vi "TouchPanel.Main.vi"(11 "VI ref":refnum<vi>) -> (1 "Canceled":bool, 2 "Label.Text":string, 3 "control used?":bool)   [LabVIEW 2016]
panel:
  out "Canceled 2":bool
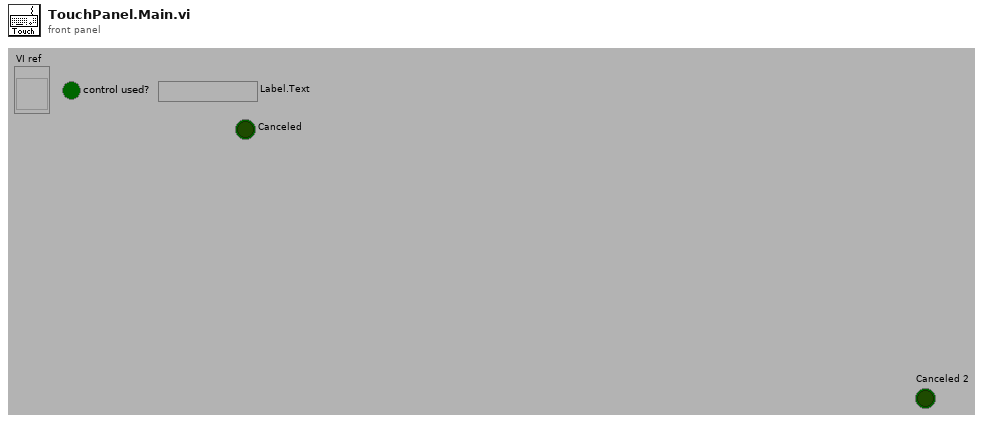
[diagram p1: front panel]
types:
  T1 = typedef "LVNumericRepresentation.ctl" = enum32{"Extended Precision", "Double Precision", "Single Precision", "Long", "Word", "Byte", "Unsigned Long", "Unsigned Word", "Unsigned Byte", "Complex Extended", "Complex Double", "Complex Single", "Quad", "Unsigned Quad", "Fixed-Point"}
  T2 = typedef "LVRowAndColumnTypeDef.ctl" = cluster{"Row":i32, "Column":i32}
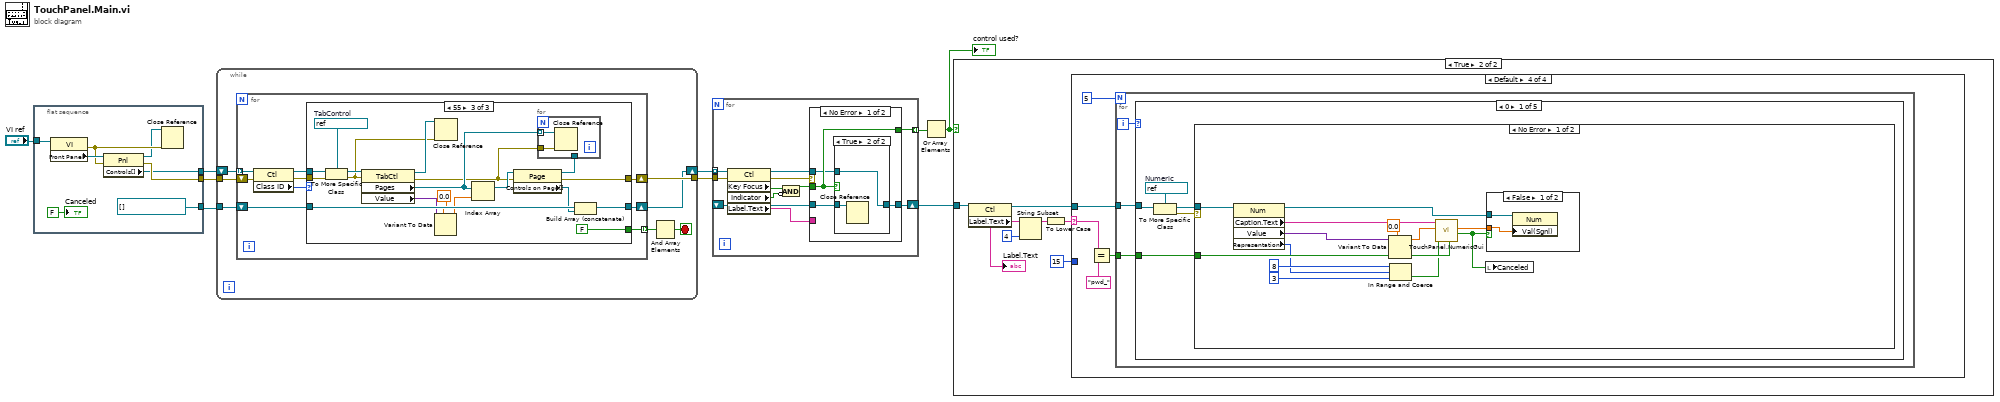
[diagram p0: block diagram]
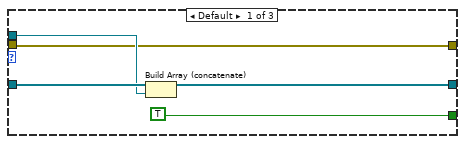
[diagram p2: hidden frame]
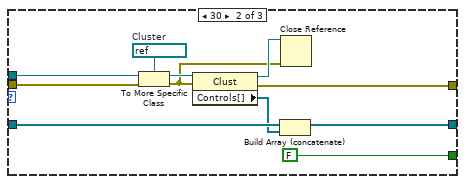
[diagram p3: hidden frame]
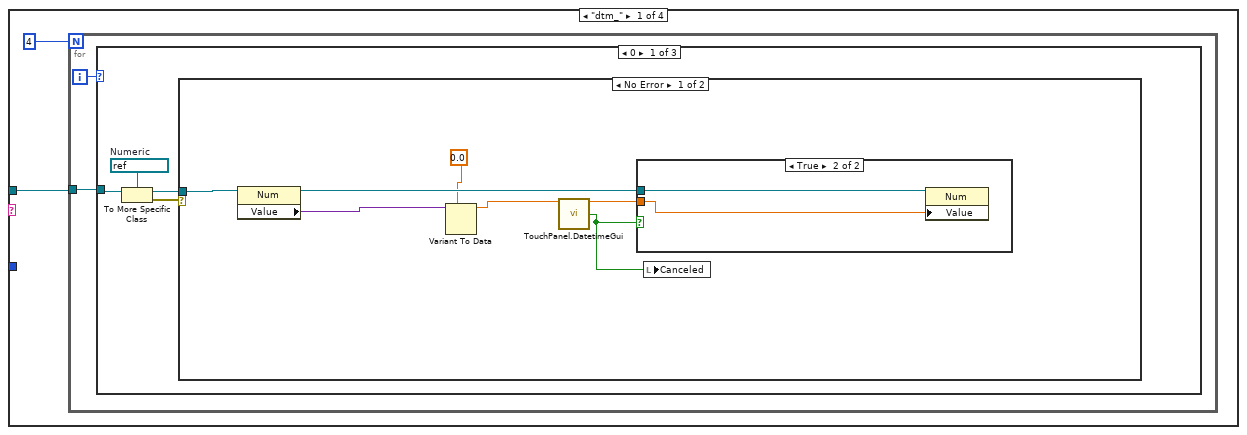
[diagram p5: hidden frame]
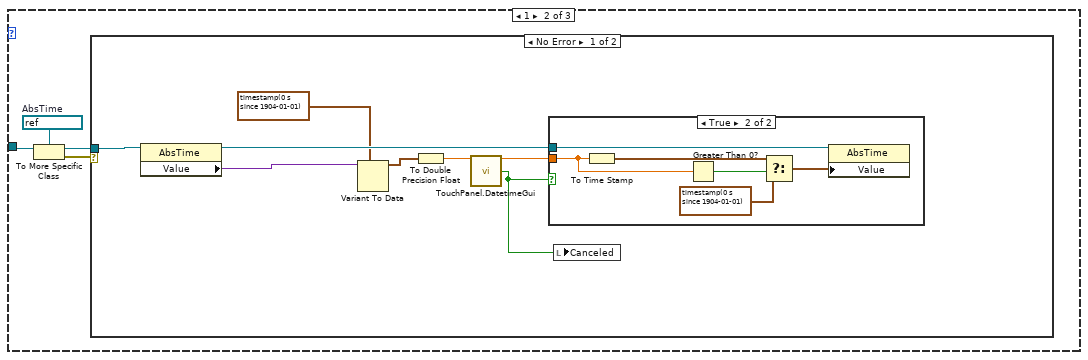
[diagram p8: hidden frame]
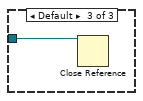
[diagram p11: hidden frame]
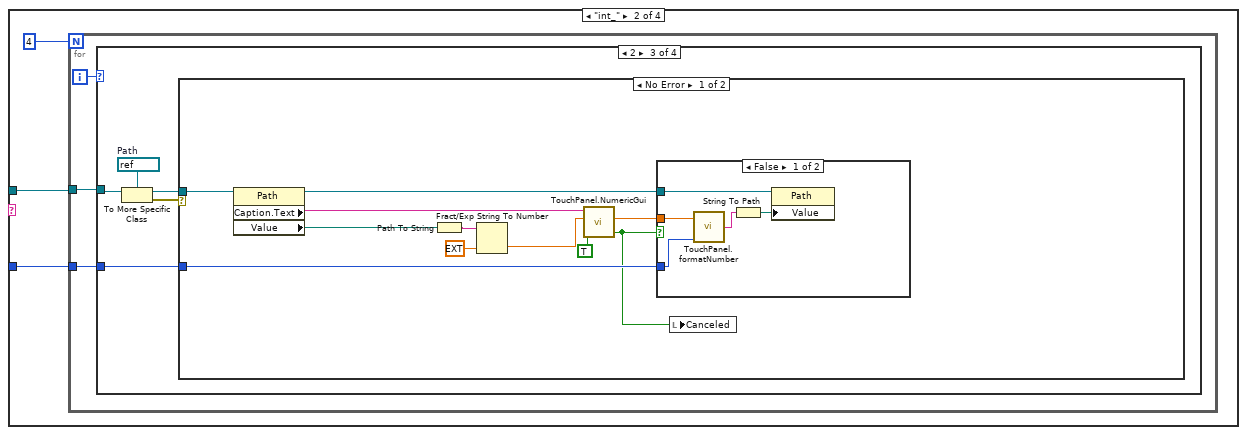
[diagram p12: hidden frame]
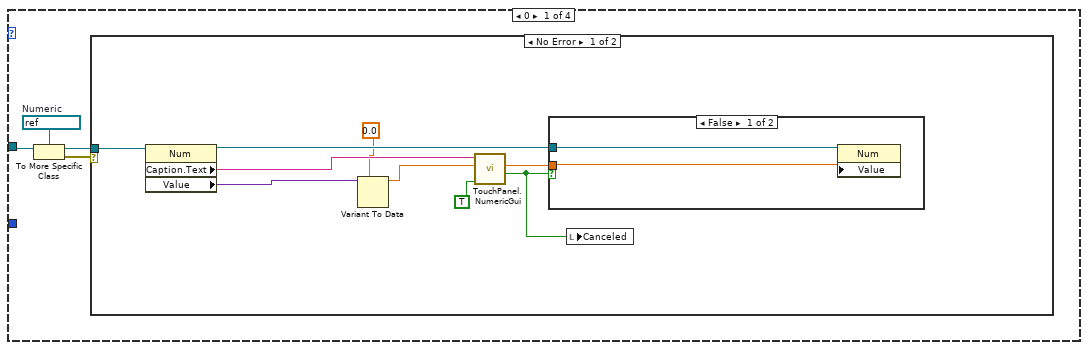
[diagram p13: hidden frame]
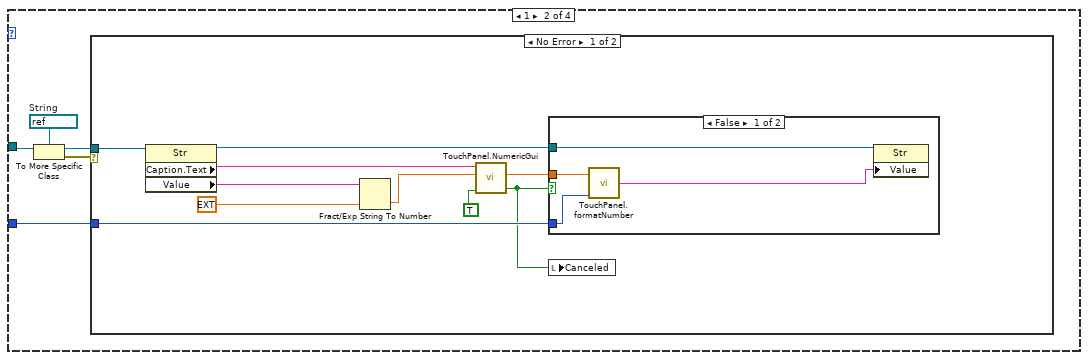
[diagram p16: hidden frame]
diagram:
  n1 = flat-sequence {
    tunnel: [w14] -> w7
    tunnel: [refnum<vi>[] []] -> w5
    tunnel: [w12] -> w4
    tunnel: "VI ref" -> [w11]
    frame #0 {
      n2 = property class="VI"(reference=w11) -> (error out=w16:errorcluster, "Front Panel"=w17:refnum<vi>)  [unwired: 1 in, 1 out]
      n3 = property class="Pnl"(reference=w17, error in=w16) -> (reference out=w15:refnum<vi>, error out=w14:errorcluster, "Controls[]"=w12:refnum<vi>[])
      n4 = Close Reference(reference=w15, error in (no error)=w16) -> ()  [unwired: 1 out]
      "Canceled" <- FALSE ("Canceled")
    }
  }
  n5 = while {
    tunnel: w7 -> [w24]
    tunnel: [w23] -> w6
    tunnel: w5 -> [w22]
    shift-right: [w20] -> w3
    shift-left: w4 -> [w21]
    stop <- w18 stop-if-true
    n6 = for {
      tunnel: w21 -> [w33] mode=indexing
      shift-right: [w27] -> w23
      shift-left: w24 -> [w32]
      shift-right: [w28] -> w20
      shift-left: w22 -> [w29]
      tunnel: [w25] -> w19 mode=indexing
      n7 = property class="Ctl"(reference=w33, error in=w32) -> (reference out=w31:refnum<vi>, error out=w30:errorcluster, "Class ID"=w26:u32)
      n8 = case shown="55" w26 {
        tunnel: w31 -> [w37 w47 w66]
        tunnel: w30 -> [w35 w46 w65]
        tunnel: w29 -> [w38 w43 w61]
        tunnel: [w36 w41 w60] -> w28
        tunnel: [w35 w40 w59] -> w27
        tunnel: [TRUE FALSE FALSE] -> w25
        frame Default {
          n9 = Build Array (concatenate)(w38, w37) -> (w36:refnum<vi>[])
        }
        frame 30 {
          w48 = refnum<vi> refnum  # Cluster
          n10 = To More Specific Class(target class=w48, reference=w47, error in=w46) -> (specific class reference=w49:refnum<vi>, error out=w44:errorcluster)
          n11 = property class="Clust"(reference=w49, error in=w44) -> (reference out=w45:refnum<vi>, error out=w40:errorcluster, "Controls[]"=w42:refnum<vi>[])
          n12 = Build Array (concatenate)(w43, w42) -> (w41:refnum<vi>[])
          n13 = Close Reference(reference=w45, error in (no error)=w44) -> ()  [unwired: 1 out]
        }
        frame 55 {
          w62 = refnum<vi> refnum  # TabControl
          n14 = To More Specific Class(target class=w62, reference=w66, error in=w65) -> (specific class reference=w67:refnum<vi>, error out=w63:errorcluster)
          n15 = property class="TabCtl"(reference=w67, error in=w63) -> (reference out=w64:refnum<vi>, error out=w51:errorcluster, "Pages"=w52:refnum<vi>[], "Value"=w57:variant)
          n16 = Variant To Data(type=0.0 ("value"), Variant=w57) -> (data=w55:dbl)  [unwired: 1 in, 1 out]
          n17 = Close Reference(reference=w64, error in (no error)=w63) -> ()  [unwired: 1 out]
          n18 = Index Array(array=w52, index=w55) -> (element=w54:refnum<vi>)
          n19 = property class="Page"(reference=w54, error in=w51) -> (reference out=w50:refnum<vi>, error out=w59:errorcluster, "Controls on Page[]"=w53:refnum<vi>[])
          n20 = for {
            tunnel: w52 -> [w69] mode=indexing
            tunnel: w51 -> [w68]
            tunnel: w50 -> [_]
            n21 = Close Reference(reference=w69, error in (no error)=w68) -> ()  [unwired: 1 out]
          }
          n22 = Build Array (concatenate)(w61, w53) -> (w60:refnum<vi>[])
        }
      }
    }
    n23 = And Array Elements(Boolean array=w19) -> (logical AND=w18:bool)
  }
  n24 = for {
    tunnel: w3 -> [w80] mode=indexing
    shift-right: [w75] -> w8
    shift-left: _ -> [w77]
    tunnel: w6 -> [w79]
    tunnel: [w74] -> w9 mode=indexing
    n25 = property class="Ctl"(reference=w80, error in=w79) -> (reference out=w78:refnum<vi>, error out=w76:errorcluster, "Key Focus"=w72:bool, "Indicator"=w71:bool, "Label.Text"=w70:string)
    n26 = Compound Arithmetic op=AND(w72, invert w71) -> (w73:bool)
    n27 = case shown="No Error" w76 {
      tunnel: w78 -> [w83 _]
      tunnel: w77 -> [w82 w90]
      tunnel: w73 -> [w84 _]
      tunnel: [w81 w90] -> w75
      tunnel: [w84 FALSE ("Key Focus")] -> w74
      tunnel: w70 -> [_ _]
      frame No Error {
        n28 = case shown="True" w84 {
          tunnel: w83 -> [w86 w87]
          tunnel: w82 -> [w85 w88]
          tunnel: [w85 w87] -> w81
          frame False {
            n29 = Close Reference(reference=w86) -> ()  [unwired: 1 in, 1 out]
          }
          frame True {
            n30 = Close Reference(reference=w88) -> ()  [unwired: 1 in, 1 out]
          }
        }
      }
      frame Error {
      }
    }
  }
  n31 = Or Array Elements(Boolean array=w9) -> (logical OR=w2:bool)
  "control used?" <- w2
  n32 = case shown="True" w2 {
    tunnel: w8 -> [_ w97]
    frame False {
    }
    frame True {
      n33 = property class="Ctl"(reference=w97) -> (reference out=w96:refnum<vi>, "Label.Text"=w91:string)  [unwired: 1 in, 1 out]
      "Label.Text" <- w91
      n34 = String Subset(string=w91, length (rest)=4 ("length (rest)")) -> (substring=w95:string)  [unwired: 1 out]
      n35 = To Lower Case(string=w95) -> (all lower case string=w93:string)
      n36 = case shown="Default" w93 {
        selector: w93 -> [_ _ _ w260]
        tunnel: w96 -> [w98 w135 w197 w262]
        tunnel: i16 15 ("significant digits (6)") -> [_ w134 w196 _]
        frame "dtm_" {
          n37 = for {
            N: 4 -> [_]
            tunnel: w98 -> [w101]
            i -> [w100]
            n38 = case shown="0" w100 {
              tunnel: w101 -> [w102 w115 w133]
              frame 0 {
                w105 = refnum<vi> refnum  # Numeric
                n39 = To More Specific Class(target class=w105, reference=w102) -> (specific class reference=w103:refnum<vi>, error out=w104:errorcluster)  [unwired: 1 in]
                n40 = case shown="No Error" w104 {
                  tunnel: w103 -> [w112 _]
                  frame No Error {
                    n41 = property class="Num"(reference=w112) -> (reference out=w111:refnum<vi>, "Value"=w110:variant)  [unwired: 1 in, 1 out]
                    n42 = Variant To Data(type=0.0 ("value"), Variant=w110) -> (data=w108:dbl)  [unwired: 1 in, 1 out]
                    n43 = call "TouchPanel.DatetimeGui.vi"("num date/time in (now)"=w108) -> ("num date/time out"=w107:dbl, "ok"=w106:bool)  [unwired: 1 in, 12 out]
                    n44 = case shown="True" w106 {
                      tunnel: w111 -> [_ w114]
                      tunnel: w107 -> [_ w113]
                      frame False {
                      }
                      frame True {
                        n45 = property class="Num"(reference=w114, "Value"=w113) -> ()  [unwired: 1 in, 2 out]
                      }
                    }
                    n46 = local write "Canceled"(w106) -> ()
                  }
                  frame Error {
                  }
                }
              }
              frame 1 {
                w118 = refnum<vi> refnum  # AbsTime
                n47 = To More Specific Class(target class=w118, reference=w115) -> (specific class reference=w116:refnum<vi>, error out=w117:errorcluster)  [unwired: 1 in]
                n48 = case shown="No Error" w117 {
                  tunnel: w116 -> [w126 _]
                  frame No Error {
                    n49 = property class="AbsTime"(reference=w126) -> (reference out=w125:refnum<vi>, "Value"=w124:variant)  [unwired: 1 in, 1 out]
                    n50 = Variant To Data(type=timestamp(0 s since 1904-01-01), Variant=w124) -> (data=w123:timestamp)  [unwired: 1 in, 1 out]
                    n51 = To Double Precision Float(number=w123) -> (double precision float=w120:dbl)
                    n52 = call "TouchPanel.DatetimeGui.vi"("num date/time in (now)"=w120) -> ("num date/time out"=w122:dbl, "ok"=w119:bool)  [unwired: 1 in, 12 out]
                    n53 = case shown="True" w119 {
                      tunnel: w125 -> [_ w132]
                      tunnel: w122 -> [_ w128]
                      frame False {
                      }
                      frame True {
                        n54 = To Time Stamp(1:w128) -> (0:w130:timestamp)
                        n55 = Greater Than 0?(x=w128) -> (x > 0?=w131:bool)
                        n56 = Select(t=w130, s=w131, f=timestamp(0 s since 1904-01-01) ("time stamp")) -> (s? t:f=w129:timestamp)
                        n57 = property class="AbsTime"(reference=w132, "Value"=w129) -> ()  [unwired: 1 in, 2 out]
                      }
                    }
                    n58 = local write "Canceled"(w119) -> ()
                  }
                  frame Error {
                  }
                }
              }
              frame Default {
                n59 = Close Reference(reference=w133) -> ()  [unwired: 1 in, 1 out]
              }
            }
          }
        }
        frame "int_" {
          n60 = for {
            N: 4 -> [_]
            tunnel: w135 -> [w139]
            tunnel: w134 -> [w137]
            i -> [w138]
            n61 = case shown="2" w138 {
              tunnel: w139 -> [w140 w157 w176 w195]
              tunnel: w137 -> [_ w155 w174 _]
              frame 0 {
                w143 = refnum<vi> refnum  # Numeric
                n62 = To More Specific Class(target class=w143, reference=w140) -> (specific class reference=w141:refnum<vi>, error out=w142:errorcluster)  [unwired: 1 in]
                n63 = case shown="No Error" w142 {
                  tunnel: w141 -> [w152 _]
                  frame No Error {
                    n64 = property class="Num"(reference=w152) -> (reference out=w151:refnum<vi>, "Caption.Text"=w149:string, "Value"=w150:variant)  [unwired: 1 in, 1 out]
                    n65 = Variant To Data(type=0.0 ("value"), Variant=w150) -> (data=w147:dbl)  [unwired: 1 in, 1 out]
                    n66 = call "TouchPanel.NumericGui.vi"("Integer (F)"=TRUE, "Numeric In"=w147, "Message In"=w149) -> ("Canceled"=w144:bool, "Numeric Out"=w146:ext)  [unwired: 3 in, 4 out]
                    n67 = case shown="False" w144 {
                      tunnel: w151 -> [w154 _]
                      tunnel: w146 -> [w153 _]
                      frame False {
                        n68 = property class="Num"(reference=w154, "Value"=w153) -> ()  [unwired: 1 in, 2 out]
                      }
                      frame True {
                      }
                    }
                    n69 = local write "Canceled"(w144) -> ()
                  }
                  frame Error {
                  }
                }
              }
              frame 1 {
                w156 = refnum<vi> refnum  # String
                n70 = To More Specific Class(target class=w156, reference=w157) -> (specific class reference=w158:refnum<vi>, error out=w159:errorcluster)  [unwired: 1 in]
                n71 = case shown="No Error" w159 {
                  tunnel: w158 -> [w169 _]
                  tunnel: w155 -> [w161 _]
                  frame No Error {
                    n72 = property class="Str"(reference=w169) -> (reference out=w168:refnum<vi>, "Caption.Text"=w165:string, "Value"=w167:string)  [unwired: 1 in, 1 out]
                    n73 = Fract/Exp String To Number(string=w167, default (0 dbl)=ext 0.0 ("default (0 DBL)")) -> (number=w164:ext)  [unwired: 1 in, 2 out]
                    n74 = call "TouchPanel.NumericGui.vi"("Integer (F)"=TRUE, "Numeric In"=w164, "Message In"=w165) -> ("Canceled"=w160:bool, "Numeric Out"=w163:ext)  [unwired: 3 in, 4 out]
                    n75 = case shown="False" w160 {
                      tunnel: w168 -> [w173 _]
                      tunnel: w163 -> [w172 _]
                      tunnel: w161 -> [w170 _]
                      frame False {
                        n76 = call "TouchPanel.formatNumber.vi"("number in"=w172, "significant digits (6)"=w170) -> ("string out"=w171:string)  [unwired: 2 in, 11 out]
                        n77 = property class="Str"(reference=w173, "Value"=w171) -> ()  [unwired: 1 in, 2 out]
                      }
                      frame True {
                      }
                    }
                    n78 = local write "Canceled"(w160) -> ()
                  }
                  frame Error {
                  }
                }
              }
              frame 2 {
                w175 = refnum<vi> refnum  # Path
                n79 = To More Specific Class(target class=w175, reference=w176) -> (specific class reference=w177:refnum<vi>, error out=w178:errorcluster)  [unwired: 1 in]
                n80 = case shown="No Error" w178 {
                  tunnel: w177 -> [w189 _]
                  tunnel: w174 -> [w180 _]
                  frame No Error {
                    n81 = property class="Path"(reference=w189) -> (reference out=w184:refnum<vi>, "Caption.Text"=w183:string, "Value"=w182:path)  [unwired: 1 in, 1 out]
                    n82 = Path To String(path=w182) -> (string=w188:string)
                    n83 = Fract/Exp String To Number(string=w188, default (0 dbl)=ext 0.0 ("default (0 DBL)")) -> (number=w186:ext)  [unwired: 1 in, 2 out]
                    n84 = call "TouchPanel.NumericGui.vi"("Integer (F)"=TRUE, "Numeric In"=w186, "Message In"=w183) -> ("Canceled"=w179:bool, "Numeric Out"=w185:ext)  [unwired: 3 in, 4 out]
                    n85 = case shown="False" w179 {
                      tunnel: w184 -> [w194 _]
                      tunnel: w185 -> [w193 _]
                      tunnel: w180 -> [w190 _]
                      frame False {
                        n86 = call "TouchPanel.formatNumber.vi"("number in"=w193, "significant digits (6)"=w190) -> ("string out"=w192:string)  [unwired: 2 in, 11 out]
                        n87 = String To Path(string=w192) -> (path=w191:path)
                        n88 = property class="Path"(reference=w194, "Value"=w191) -> ()  [unwired: 1 in, 2 out]
                      }
                      frame True {
                      }
                    }
                    n89 = local write "Canceled"(w179) -> ()
                  }
                  frame Error {
                  }
                }
              }
              frame Default {
                n90 = Close Reference(reference=w195) -> ()  [unwired: 1 in, 1 out]
              }
            }
          }
        }
        frame "num_" {
          n91 = for {
            N: 4 -> [_]
            tunnel: w197 -> [w201]
            tunnel: w196 -> [w199]
            i -> [w200]
            n92 = case shown="1" w200 {
              tunnel: w201 -> [w202 w222 w240 w258]
              tunnel: w199 -> [_ w220 w238 _]
              frame 0 {
                w205 = refnum<vi> refnum  # Numeric
                n93 = To More Specific Class(target class=w205, reference=w202) -> (specific class reference=w203:refnum<vi>, error out=w204:errorcluster)  [unwired: 1 in]
                n94 = case shown="No Error" w204 {
                  tunnel: w203 -> [w217 _]
                  frame No Error {
                    n95 = property class="Num"(reference=w217) -> (reference out=w216:refnum<vi>, "Caption.Text"=w214:string, "Value"=w215:variant, "Representation"=w210:T1)  [unwired: 1 in, 1 out]
                    n96 = Variant To Data(type=0.0 ("value"), Variant=w215) -> (data=w212:dbl)  [unwired: 1 in, 1 out]
                    n97 = In Range and Coerce(upper limit=u32 8, x=w210, lower limit=u32 3 ("upper limit")) -> (In Range?=w209:bool)  [unwired: 1 out]
                    n98 = call "TouchPanel.NumericGui.vi"("Integer (F)"=w209, "Numeric In"=w212, "Message In"=w214) -> ("Canceled"=w206:bool, "Numeric Out"=w211:ext)  [unwired: 3 in, 4 out]
                    n99 = case shown="False" w206 {
                      tunnel: w216 -> [w219 _]
                      tunnel: w211 -> [w218 _]
                      frame False {
                        n100 = property class="Num"(reference=w219, "Value"=w218) -> ()  [unwired: 1 in, 2 out]
                      }
                      frame True {
                      }
                    }
                    n101 = local write "Canceled"(w206) -> ()
                  }
                  frame Error {
                  }
                }
              }
              frame 1 {
                w221 = refnum<vi> refnum  # String
                n102 = To More Specific Class(target class=w221, reference=w222) -> (specific class reference=w223:refnum<vi>, error out=w224:errorcluster)  [unwired: 1 in]
                n103 = case shown="No Error" w224 {
                  tunnel: w223 -> [w233 _]
                  tunnel: w220 -> [w226 _]
                  frame No Error {
                    n104 = property class="Str"(reference=w233) -> (reference out=w232:refnum<vi>, "Caption.Text"=w229:string, "Value"=w231:string)  [unwired: 1 in, 1 out]
                    n105 = Fract/Exp String To Number(string=w231, default (0 dbl)=ext 0.0 ("default (0 DBL)")) -> (number=w228:ext)  [unwired: 1 in, 2 out]
                    n106 = call "TouchPanel.NumericGui.vi"("Numeric In"=w228, "Message In"=w229) -> ("Canceled"=w225:bool, "Numeric Out"=w227:ext)  [unwired: 4 in, 4 out]
                    n107 = case shown="False" w225 {
                      tunnel: w232 -> [w237 _]
                      tunnel: w227 -> [w236 _]
                      tunnel: w226 -> [w234 _]
                      frame False {
                        n108 = call "TouchPanel.formatNumber.vi"("number in"=w236, "significant digits (6)"=w234) -> ("string out"=w235:string)  [unwired: 2 in, 11 out]
                        n109 = property class="Str"(reference=w237, "Value"=w235) -> ()  [unwired: 1 in, 2 out]
                      }
                      frame True {
                      }
                    }
                    n110 = local write "Canceled"(w225) -> ()
                  }
                  frame Error {
                  }
                }
              }
              frame 2 {
                w239 = refnum<vi> refnum  # Path
                n111 = To More Specific Class(target class=w239, reference=w240) -> (specific class reference=w241:refnum<vi>, error out=w242:errorcluster)  [unwired: 1 in]
                n112 = case shown="No Error" w242 {
                  tunnel: w241 -> [w252 _]
                  tunnel: w238 -> [w244 _]
                  frame No Error {
                    n113 = property class="Path"(reference=w252) -> (reference out=w247:refnum<vi>, "Caption.Text"=w246:string, "Value"=w245:path)  [unwired: 1 in, 1 out]
                    n114 = Path To String(path=w245) -> (string=w251:string)
                    n115 = Fract/Exp String To Number(string=w251, default (0 dbl)=ext 0.0 ("default (0 DBL)")) -> (number=w249:ext)  [unwired: 1 in, 2 out]
                    n116 = call "TouchPanel.NumericGui.vi"("Numeric In"=w249, "Message In"=w246) -> ("Canceled"=w243:bool, "Numeric Out"=w248:ext)  [unwired: 4 in, 4 out]
                    n117 = local write "Canceled"(w243) -> ()
                    n118 = case shown="False" w243 {
                      tunnel: w247 -> [w257 _]
                      tunnel: w248 -> [w256 _]
                      tunnel: w244 -> [w253 _]
                      frame False {
                        n119 = call "TouchPanel.formatNumber.vi"("number in"=w256, "significant digits (6)"=w253) -> ("string out"=w255:string)  [unwired: 2 in, 11 out]
                        n120 = String To Path(string=w255) -> (path=w254:path)
                        n121 = property class="Path"(reference=w257, "Value"=w254) -> ()  [unwired: 1 in, 2 out]
                      }
                      frame True {
                      }
                    }
                  }
                  frame Error {
                  }
                }
              }
              frame Default {
                n122 = Close Reference(reference=w258) -> ()  [unwired: 1 in, 1 out]
              }
            }
          }
        }
        frame Default {
          n123 = Equal?(x=w260, y="pwd_") -> (x = y?=w261:bool)
          n124 = for {
            N: 5 -> [_]
            tunnel: w262 -> [w266]
            tunnel: w261 -> [w264]
            i -> [w265]
            n125 = case shown="0" w265 {
              tunnel: w266 -> [w268 w289 w304 w320 w367]
              tunnel: w264 -> [w267 w287 w302 w319 _]
              frame 0 {
                w271 = refnum<vi> refnum  # Numeric
                n126 = To More Specific Class(target class=w271, reference=w268) -> (specific class reference=w269:refnum<vi>, error out=w270:errorcluster)  [unwired: 1 in]
                n127 = case shown="No Error" w270 {
                  tunnel: w269 -> [w274 _]
                  tunnel: w267 -> [w279 _]
                  frame No Error {
                    n128 = property class="Num"(reference=w274) -> (reference out=w273:refnum<vi>, "Caption.Text"=w283:string, "Value"=w284:variant, "Representation"=w276:T1)  [unwired: 1 in, 1 out]
                    n129 = Variant To Data(type=0.0 ("value"), Variant=w284) -> (data=w281:dbl)  [unwired: 1 in, 1 out]
                    n130 = In Range and Coerce(upper limit=u32 8, x=w276, lower limit=u32 3 ("upper limit")) -> (In Range?=w275:bool)  [unwired: 1 out]
                    n131 = call "TouchPanel.NumericGui.vi"("Password Display (F)"=w279, "Integer (F)"=w275, "Numeric In"=w281, "Message In"=w283) -> ("Canceled"=w272:bool, "Numeric Out"=w280:ext)  [unwired: 2 in, 4 out]
                    n132 = local write "Canceled"(w272) -> ()
                    n133 = case shown="False" w272 {
                      tunnel: w273 -> [w286 _]
                      tunnel: w280 -> [w285 _]
                      frame False {
                        n134 = property class="Num"(reference=w286, "Val(Sgnl)"=w285) -> ()  [unwired: 1 in, 2 out]
                      }
                      frame True {
                      }
                    }
                  }
                  frame Error {
                  }
                }
              }
              frame 1 {
                w288 = refnum<vi> refnum  # String
                n135 = To More Specific Class(target class=w288, reference=w289) -> (specific class reference=w290:refnum<vi>, error out=w291:errorcluster)  [unwired: 1 in]
                n136 = case shown="No Error" w291 {
                  tunnel: w290 -> [w299 _]
                  tunnel: w287 -> [w294 _]
                  frame No Error {
                    n137 = property class="Str"(reference=w299) -> (reference out=w298:refnum<vi>, "Caption.Text"=w296:string, "Value"=w297:string, "Limit To Single Line?"=w293:bool)  [unwired: 1 in, 1 out]
                    n138 = call "TouchPanel.AlphanumericGui.vi"("Password Display (F)"=w294, "Limit to single line (T)"=w293, "String In"=w297, "Message In"=w296) -> ("Canceled"=w292:bool, "String Out"=w295:string)  [unwired: 1 in, 5 out]
                    n139 = local write "Canceled"(w292) -> ()
                    n140 = case shown="False" w292 {
                      tunnel: w298 -> [w301 _]
                      tunnel: w295 -> [w300 _]
                      frame False {
                        n141 = property class="Str"(reference=w301, "Val(Sgnl)"=w300) -> ()  [unwired: 1 in, 2 out]
                      }
                      frame True {
                      }
                    }
                  }
                  frame Error {
                  }
                }
              }
              frame 2 {
                w303 = refnum<vi> refnum  # Path
                n142 = To More Specific Class(target class=w303, reference=w304) -> (specific class reference=w305:refnum<vi>, error out=w306:errorcluster)  [unwired: 1 in]
                n143 = case shown="No Error" w306 {
                  tunnel: w305 -> [w315 _]
                  tunnel: w302 -> [w308 _]
                  frame No Error {
                    n144 = property class="Path"(reference=w315) -> (reference out=w314:refnum<vi>, "Caption.Text"=w311:string, "Value"=w313:path)  [unwired: 1 in, 1 out]
                    n145 = Path To String(path=w313) -> (string=w310:string)
                    n146 = call "TouchPanel.AlphanumericGui.vi"("Password Display (F)"=w308, "String In"=w310, "Message In"=w311) -> ("Canceled"=w307:bool, "String Out"=w309:string)  [unwired: 2 in, 5 out]
                    n147 = String To Path(string=w309) -> (path=w312:path)
                    n148 = case shown="False" w307 {
                      tunnel: w314 -> [w317 _]
                      tunnel: w312 -> [w316 _]
                      frame False {
                        n149 = property class="Path"(reference=w317, "Val(Sgnl)"=w316) -> ()  [unwired: 1 in, 2 out]
                      }
                      frame True {
                      }
                    }
                    n150 = local write "Canceled"(w307) -> ()
                  }
                  frame Error {
                  }
                }
              }
              frame 3 {
                n151 = To More Specific Class(target class=refnum<vi> refnum ("Table"), reference=w320) -> (specific class reference=w321:refnum<vi>, error out=w322:errorcluster)  [unwired: 1 in]
                n152 = case shown="No Error" w322 {
                  tunnel: w321 -> [w334 _]
                  tunnel: w319 -> [w332 _]
                  frame No Error {
                    n153 = property class="Tbl (strict)" props=["Row Headers[]", "Column Headers[]", "Caption", "Text", "Value", "EditPos"](reference=w334) -> (reference out=w333:refnum<vi>, "Row Headers[]"=w330:string[], "Column Headers[]"=w329:string[], "Value"=w327:string[][], "EditPos"=w331:T2)  [unwired: 1 in, 2 out]
                    n154 = Array Size(array=w327) -> (size(s)=w326:i32[])
                    n155 = Unbundle(w331) -> ("Row"=w324:i32, "Column"=w328:i32)
                    n156 = Index Array(array=w326) -> (element=w325:i32)  [unwired: 1 in]
                    n157 = Less?(x=w324, y=w325) -> (x < y?=w323:bool)
                    n158 = case shown="True" w323 {
                      tunnel: w333 -> [_ w357]
                      tunnel: w332 -> [_ w356]
                      tunnel: w331 -> [_ w352]
                      tunnel: w330 -> [_ w350]
                      tunnel: w329 -> [_ w349]
                      tunnel: w328 -> [_ w348]
                      tunnel: w327 -> [_ w343]
                      tunnel: w324 -> [_ w342]
                      frame False {
                      }
                      frame True {
                        n159 = Index Array(array=w349, index=w348) -> (element=w346:string)
                        n160 = Index Array(array=w350, index=w342) -> (element=w347:string)
                        n161 = Index Array(array=w343, index (row)=w342, index (col)=w348) -> (element=w355:string)
                        n162 = Concatenate Strings(w347, " - ", w346) -> (w344:string)
                        n163 = Fract/Exp String To Number(string=w355, default (0 dbl)=ext 0.0 ("default (0 DBL)")) -> (number=w353:ext)  [unwired: 1 in, 2 out]
                        n164 = call "TouchPanel.NumericGui.vi"("Password Display (F)"=w356, "empty visible (F)"=TRUE, "Numeric In"=w353, "Message In"=w344) -> ("Canceled"=w335:bool, "Numeric Out"=w341:ext)  [unwired: 2 in, 4 out]
                        n165 = Number To Fractional String(number=w341, precision (6)=i16 9) -> (F-format string=w339:string)  [unwired: 1 in, 1 out]
                        n166 = Not A Number/Path/Refnum?(number/path/refnum=w341) -> (NaN/Path/Refnum?=w340:bool)
                        n167 = local write "Canceled"(w335) -> ()
                        n168 = Select(t="", s=w340, f=w339) -> (s? t:f=w337:string)
                        n169 = case shown="False" w335 {
                          tunnel: w357 -> [w366 _]
                          tunnel: w337 -> [w359 _]
                          tunnel: w352 -> [w358 _]
                          frame False {
                            n170 = property class="Tbl (strict)"(reference=w366) -> (reference out=w365:refnum<vi>, error out=w364:errorcluster, "Value"=w363:string[][])  [unwired: 1 in]
                            n171 = Unbundle(w358) -> ("Row"=w361:i32, "Column"=w360:i32)
                            n172 = Replace Array Subset(array=w363, new element=w359, index (row)=w361, index (col)=w360) -> (w362:string[][])
                            n173 = property class="Tbl (strict)"(reference=w365, error in=w364, "Val(Sgnl)"=w362) -> ()  [unwired: 2 out]
                          }
                          frame True {
                          }
                        }
                      }
                    }
                  }
                  frame Error {
                  }
                }
              }
              frame Default {
                n174 = Close Reference(reference=w367) -> ()  [unwired: 1 in, 1 out]
              }
            }
          }
        }
      }
    }
  }
